vi "Set_SP.vi"(8 "error in":errorcluster, 10 "SP /Ohms":dbl=1.0, 11 "VISA name":refnum<visa-resource-name>) -> (0 "error out":errorcluster, 1 "valid":bool, 2 "output":T1 {"SP read /Ohms" format="%#.6g"}, 3 "VISA out":refnum<visa-resource-name>)   [LabVIEW 2018, in "QR-10x.lvlib"]
uses:
  QR-10x.lvlib
panel:
  out "buffer":string
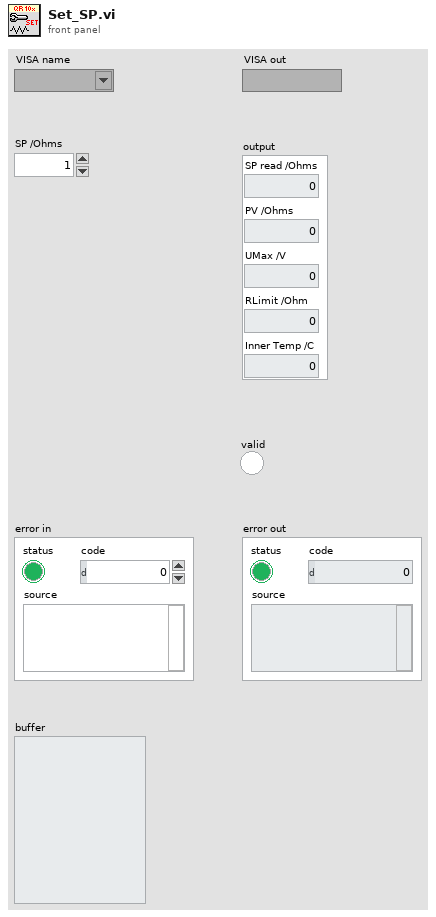
[diagram p1: front panel]
types:
  T1 = cluster{"SP read /Ohms":dbl, "PV /Ohms":dbl, "UMax /V":dbl, "RLimit /Ohm":dbl, "Inner Temp /C":dbl}
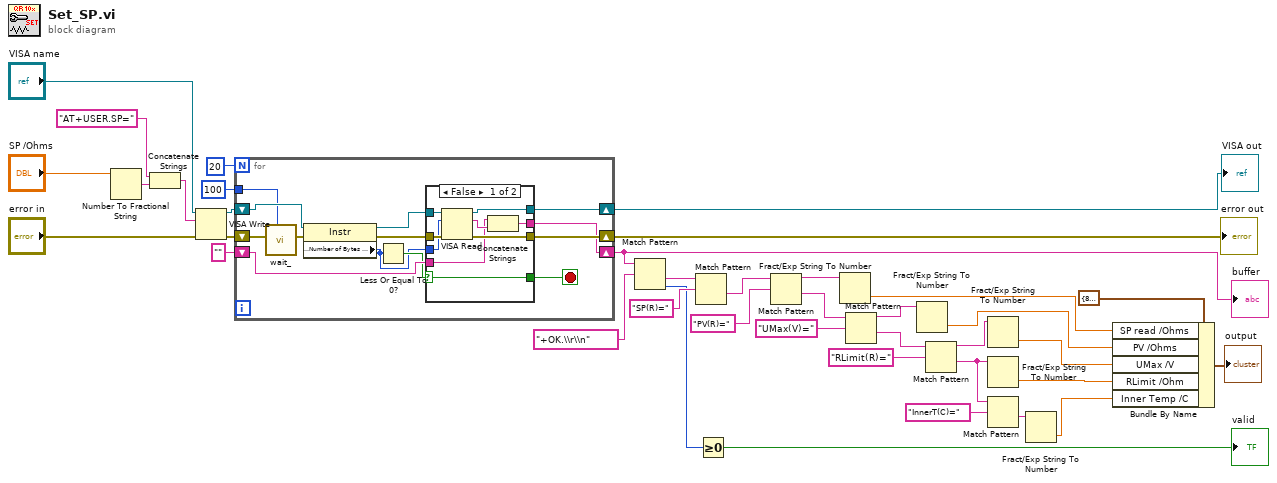
[diagram p0: block diagram]
diagram:
  n1 = Number To Fractional String(number="SP /Ohms") -> (F-format string=w16:string)  [unwired: 3 in]
  n2 = Concatenate Strings("AT+USER.SP=" ("write buffer"), w16) -> (w33:string)
  n3 = VISA Write(VISA resource name="VISA name", write buffer=w33, error in (no error)="error in") -> (VISA resource name out=w38:refnum<visa-resource-name>, error out=w32:errorcluster)  [unwired: 1 out]
  n4 = for {
    N: 20 -> [_]
    shift-right: [w47] -> w18
    shift-left: w38 -> [w51]
    shift-right: [w48] -> w17
    shift-left: w32 -> [w41]
    shift-right: [w46] -> w14
    shift-left: "" -> [w45]
    tunnel: u32 100 ("milliseconds to wait") -> [w39]
    stop <- w44 stop-if-true
    n5 = call "wait_.vi"("milliseconds to wait"=w39, "error in"=w41) -> ("error out"=w40:errorcluster)  [unwired: 9 in]
    n6 = property class="Instr"(reference=w51, error in=w40) -> (reference out=w49:refnum<visa-resource-name>, error out=w50:errorcluster, "Serial Settings:Number of Bytes at Serial Port"=w42:u32)
    n7 = Less Or Equal To 0?(x=w42) -> (x <= 0?=w43:bool)
    n8 = case shown="False" w43 {
      selector: w43 -> [w53 w61]
      tunnel: w50 -> [w60 w64]
      tunnel: w49 -> [w59 w63]
      tunnel: [w58 w64] -> w48
      tunnel: [w57 w63] -> w47
      tunnel: [w55 w62] -> w46
      tunnel: w45 -> [w54 w62]
      tunnel: [w53 w61] -> w44
      tunnel: w42 -> [w52 _]
      frame False {
        n9 = VISA Read(VISA resource name=w59, byte count=w52, error in (no error)=w60) -> (VISA resource name out=w57:refnum<visa-resource-name>, read buffer=w56:string, error out=w58:errorcluster)  [unwired: 1 out]
        n10 = Concatenate Strings(w54, w56) -> (w55:string)
      }
      frame True {
      }
    }
  }
  "buffer" <- w14
  "error out" <- w17
  "VISA out" <- w18
  n11 = Match Pattern(string=w14, regular expression="+OK.\\r\\n") -> (after substring=w22:string, offset past match=w13:i32)  [unwired: 1 in, 2 out]
  n12 = Match Pattern(string=w22, regular expression="SP(R)=") -> (after substring=w20:string)  [unwired: 1 in, 3 out]
  n13 = Greater Or Equal To 0?(x=w13) -> (x >= 0?=→"valid":bool)
  n14 = Match Pattern(string=w20, regular expression="PV(R)=") -> (before substring=w25:string, after substring=w28:string)  [unwired: 1 in, 2 out]
  n15 = Fract/Exp String To Number(string=w25) -> (number=w7:dbl)  [unwired: 3 in, 1 out]
  n16 = Match Pattern(string=w28, regular expression="UMax(V)=") -> (before substring=w24:string, after substring=w26:string)  [unwired: 1 in, 2 out]
  n17 = Fract/Exp String To Number(string=w24) -> (number=w6:dbl)  [unwired: 3 in, 1 out]
  n18 = Match Pattern(string=w26, regular expression="RLimit(R)=") -> (before substring=w23:string, after substring=w11:string)  [unwired: 1 in, 2 out]
  n19 = Fract/Exp String To Number(string=w23) -> (number=w5:dbl)  [unwired: 3 in, 1 out]
  n20 = Fract/Exp String To Number(string=w11) -> (number=w4:dbl)  [unwired: 3 in, 1 out]
  n21 = Match Pattern(string=w11, regular expression="InnerT(C)=") -> (after substring=w9:string)  [unwired: 1 in, 3 out]
  n22 = Fract/Exp String To Number(string=w9) -> (number=w3:dbl)  [unwired: 3 in, 1 out]
  n23 = Bundle By Name(cluster=T1 {"SP read /Ohms"=88.98, "PV /Ohms"=88.974, "UMax /V"=8.4, "RLimit /Ohm"=0.01, "Inner Temp /C"=0.01} ("Cluster"), "SP read /Ohms"=w7, "PV /Ohms"=w6, "UMax /V"=w5, "RLimit /Ohm"=w4, "Inner Temp /C"=w3) -> (→"output":T1)
